vi "audio output.vi"(0 "notifier":refnum<notifier>) -> ()   [LabVIEW 2009]
uses:
  <vilib>/sound2/lvsound2.llb/Sound Data Format.ctl
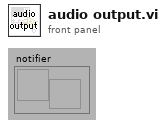
[diagram p1: front panel]
types:
  T1 = typedef "Sound Data Format.ctl" = cluster{"sample rate (S/s)":dbl, "number of channels":i32, "bits per sample":i32}
  T2 = enum16{"Buffer and play", "Update", "Pause", "End"}
  T3 = typedef "Sound Output Task ID.ctl" = u32
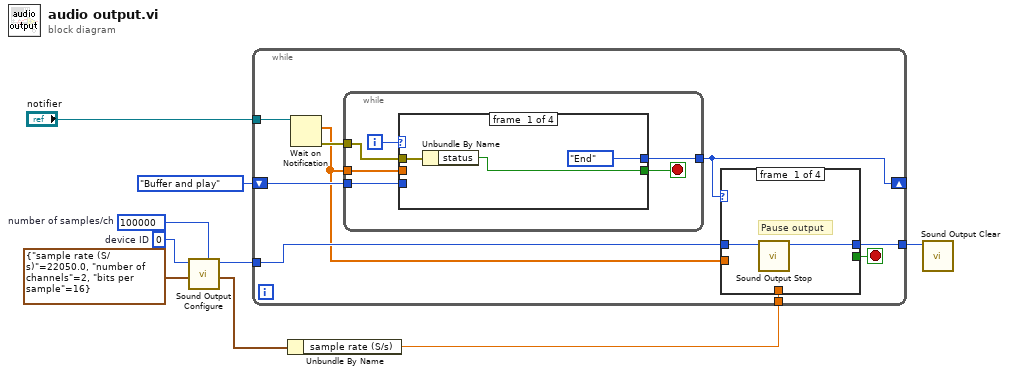
[diagram p0: block diagram]
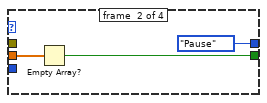
[diagram p2: hidden frame]
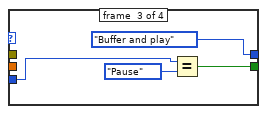
[diagram p3: hidden frame]
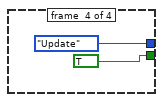
[diagram p4: hidden frame]
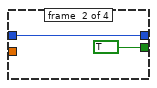
[diagram p5: hidden frame]
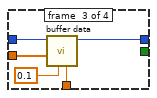
[diagram p6: hidden frame]
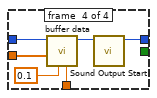
[diagram p7: hidden frame]
diagram:
  w3 = 100000  # number of samples/ch
  w2 = T1 {"sample rate (S/s)"=22050.0, "number of channels"=2, "bits per sample"=16} ("sound format")
  w4 = u32 0  # device ID
  n1 = call <vilib>:"Sound Output Configure.vi"("number of samples/ch"=w3, "sound format"=w2, "device ID"=w4) -> ("task ID"=w7:T3)  [unwired: 7 in, 1 out]
  n2 = Unbundle By Name(w2) -> ("sample rate (S/s)"=w1:dbl)
  n3 = while {
    tunnel: "notifier" -> [w17]
    tunnel: w7 -> [w16]
    tunnel: [w15] -> w8
    shift-right: [w11] -> _
    shift-left: T2."Buffer and play" -> [w12]
    tunnel: w1 -> [w9]
    stop <- w14 stop-if-true
    n4 = Wait on Notification(notifier=w17) -> (notification=w10:sgl[], error out=w13:errorcluster)  [unwired: 3 in, 2 out]
    n5 = while {
      tunnel: w13 -> [w23]
      tunnel: w10 -> [w21]
      tunnel: w12 -> [w20]
      tunnel: [w19] -> w11
      i -> [w22]
      stop <- w18 stop-if-true
      n6 = case shown="0" w22 {
        tunnel: w23 -> [w25 _ _ _]
        tunnel: w21 -> [_ w27 _ _]
        tunnel: w20 -> [_ _ w31 _]
        tunnel: [T2."End" T2."Pause" T2."Buffer and play" T2."Update"] -> w19
        tunnel: [w24 w28 w30 TRUE ("empty?")] -> w18
        frame #0 {
          n7 = Unbundle By Name(w25) -> ("status"=w24:bool)
        }
        frame #1 {
          n8 = Empty Array?(array=w27) -> (empty?=w28:bool)
        }
        frame #2 {
          n9 = Equal?(x=w31, y=T2."Pause") -> (x = y?=w30:bool)
        }
        frame #3 {
        }
      }
    }
    n10 = case shown="\"Update\"" w11 {
      tunnel: w16 -> [w37 w39 w44 w49]
      tunnel: [w36 w39 w43 w50] -> w15
      tunnel: [_ TRUE _ _] -> w14
      tunnel: w10 -> [_ _ w41 w47]
      tunnel: w9 -> [_ _ w42 w46]
      frame #0 {
        # "Pause output"
        n11 = call <vilib>:"Sound Output Stop.vi"("task ID"=w37) -> ("task ID out"=w36:T3)  [unwired: 9 in, 1 out]
      }
      frame #1 {
      }
      frame #2 {
        n12 = call "buffer data.vi"("Samples/second"=w42, "buffer time (s)"=0.1, "Data to write"=w41, "task ID"=w44) -> ("task ID out"=w43:T3)  [unwired: 6 in, 1 out]
      }
      frame #3 {
        n13 = call "buffer data.vi"("Samples/second"=w46, "buffer time (s)"=0.1, "Data to write"=w47, "task ID"=w49) -> ("task ID out"=w48:T3)  [unwired: 6 in, 1 out]
        n14 = call <vilib>:"Sound Output Start.vi"("task ID"=w48) -> ("task ID out"=w50:T3)  [unwired: 9 in, 1 out]
      }
    }
  }
  n15 = call <vilib>:"Sound Output Clear.vi"("task ID"=w8) -> ()  [unwired: 10 in, 1 out]
